vi "로봇대회1.vi"() -> ()   [LabVIEW 2010]
uses:
  <vilib>/NXT/Subs/MotorOutput.ctl
  <vilib>/NXT/Block Support/NXT_InputPort.ctl
  <vilib>/NXT/Dual Mode Library/Sensors/Sonar_cm.vi
  <vilib>/NXT/Dual Mode Library/Motors/MotorOn.vi
  <vilib>/NXT/Dual Mode Library/Sensors/Light_On.vi
  <vilib>/NXT/Dual Mode Library/Motors/MotorReverse.vi
  <vilib>/NXT/Dual Mode Library/Waits/Wait_Rotation.vi
  <vilib>/NXT/Dual Mode Library/Waits/Wait_Num.vi
panel:
  in  "정지":bool
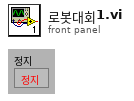
[diagram p1: front panel]
types:
  T1 = typedef "MotorOutput.ctl" = u8
  T2 = typedef "NXT_InputPort.ctl" = u8
  T3 = typedef "LVHSConnector.ctl" = cluster{"error":errorcluster, "address":string, "NXT #":i32, "Show Error":bool, "Connection":u16}
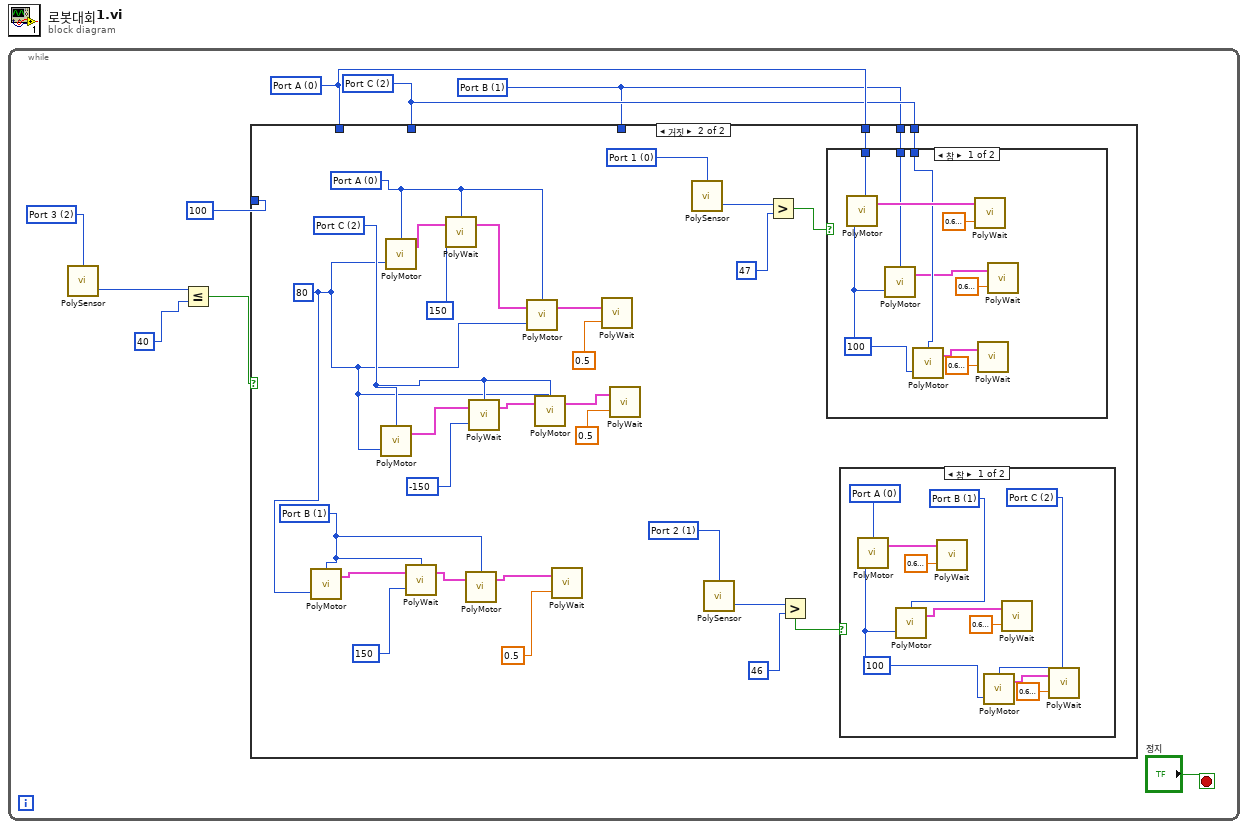
[diagram p0: block diagram]
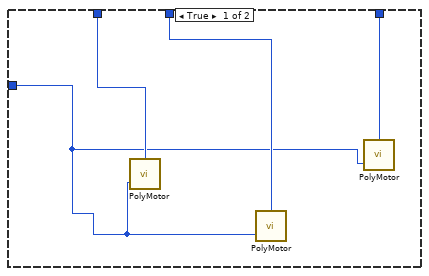
[diagram p2: hidden frame]
diagram:
  n1 = while {
    stop <- "정지" stop-if-true
    w1 = T1 1 items=["Port A", "Port B", "Port C", "All Ports"] ("Output Port (All Ports)")
    w2 = T1 2 items=["Port A", "Port B", "Port C", "All Ports"] ("Output Port (All Ports)")
    w3 = T1 0 items=["Port A", "Port B", "Port C", "All Ports"] ("Output Port (All Ports)")
    w6 = T2 2 items=["Port 1", "Port 2", "Port 3", "Port 4"] ("Input Port")
    n2 = call-poly <vilib>:"PolySensor.vi"("Port (Port 4)"=w6) -> ("Distance (cm)"=w4:i16)  [unwired: 2 in, 1 out]
    n3 = Less Or Equal?(x=w4, y=40) -> (x <= y?=w7:bool)
    n4 = case shown="거짓" w7 {
      tunnel: w3 -> [w13 _]
      tunnel: w2 -> [w12 _]
      tunnel: 100 ("Power (75)") -> [w10 _]
      tunnel: w1 -> [w11 _]
      tunnel: w3 -> [_ w23]
      tunnel: w2 -> [_ w22]
      tunnel: w1 -> [_ w21]
      frame True {
        n5 = call-poly <vilib>:"PolyMotor.vi"("Power (75)"=w10, "Output Port (All Ports)"=w13) -> ()  [unwired: 2 in, 1 out]
        n6 = call-poly <vilib>:"PolyMotor.vi"("Power (75)"=w10, "Output Port (All Ports)"=w12) -> ()  [unwired: 2 in, 1 out]
        n7 = call-poly <vilib>:"PolyMotor.vi"("Power (75)"=w10, "Output Port (All Ports)"=w11) -> ()  [unwired: 2 in, 1 out]
      }
      frame False {
        w14 = T1 1 items=["Port A", "Port B", "Port C", "All Ports"] ("Output Port (All Ports)")
        w25 = T2 1 items=["Port 1", "Port 2", "Port 3", "Port 4"] ("Input Port")
        w24 = T2 0 items=["Port 1", "Port 2", "Port 3", "Port 4"] ("Input Port")
        w17 = 80 ("Power (75)")
        w33 = T1 2 items=["Port A", "Port B", "Port C", "All Ports"] ("Output Port (All Ports)")
        w34 = T1 0 items=["Port A", "Port B", "Port C", "All Ports"] ("Output Port (All Ports)")
        n8 = call-poly <vilib>:"PolyMotor.vi"("Power (75)"=w17, "Output Port (All Ports)"=w14) -> ("NXT"=w18:T3)  [unwired: 2 in]
        n9 = call-poly <vilib>:"PolyMotor.vi"("Power (75)"=w17, "Output Port (All Ports)"=w33) -> ("NXT"=w42:T3)  [unwired: 2 in]
        n10 = call-poly <vilib>:"PolyMotor.vi"("Power (75)"=w17, "Output Port (All Ports)"=w34) -> ("NXT"=w43:T3)  [unwired: 2 in]
        n11 = call-poly <vilib>:"PolyWait.vi"("Position Change (180)"=150, "NXT"=w18, "Port (Port A)"=w14) -> ("NXT"=w19:T3)  [unwired: 1 in]
        n12 = call-poly <vilib>:"PolyWait.vi"("Position Change (180)"=150, "NXT"=w43, "Port (Port A)"=w34) -> ("NXT"=w39:T3)  [unwired: 1 in]
        n13 = call-poly <vilib>:"PolyMotor.vi"("NXT"=w19, "Output Port (All Ports)"=w14) -> ("NXT"=w20:T3)  [unwired: 2 in]
        n14 = call-poly <vilib>:"PolyWait.vi"("Position Change (180)"=-150, "NXT"=w42, "Port (Port A)"=w33) -> ("NXT"=w36:T3)  [unwired: 1 in]
        n15 = call-poly <vilib>:"PolyMotor.vi"("Power (75)"=w17, "NXT"=w39, "Output Port (All Ports)"=w34) -> ("NXT"=w38:T3)  [unwired: 1 in]
        n16 = call-poly <vilib>:"PolyMotor.vi"("Power (75)"=w17, "NXT"=w36, "Output Port (All Ports)"=w33) -> ("NXT"=w35:T3)  [unwired: 1 in]
        n17 = call-poly <vilib>:"PolyWait.vi"("Time (sec)"=sgl 0.5 ("Time (1 sec)"), "NXT"=w20) -> ()  [unwired: 2 in, 1 out]
        n18 = call-poly <vilib>:"PolyWait.vi"("Time (sec)"=sgl 0.5 ("Time (1 sec)"), "NXT"=w38) -> ()  [unwired: 2 in, 1 out]
        n19 = call-poly <vilib>:"PolyWait.vi"("Time (sec)"=sgl 0.5 ("Time (1 sec)"), "NXT"=w35) -> ()  [unwired: 2 in, 1 out]
        n20 = call-poly <vilib>:"PolySensor.vi"("Port (Port 3)"=w24) -> ("Scaled Value"=w28:i16)  [unwired: 2 in, 1 out]
        n21 = call-poly <vilib>:"PolySensor.vi"("Port (Port 3)"=w25) -> ("Scaled Value"=w31:i16)  [unwired: 2 in, 1 out]
        n22 = Greater?(x=w28, y=47) -> (0:w26:bool)
        n23 = Greater?(x=w31, y=46) -> (0:w29:bool)
        n24 = case shown="참" w26 {
          tunnel: w23 -> [w49 _]
          tunnel: w22 -> [w48 _]
          tunnel: w21 -> [w44 _]
          frame True {
            w45 = 100 ("Power (75)")
            n25 = call-poly <vilib>:"PolyMotor.vi"("Power (75)"=w45, "Output Port (All Ports)"=w49) -> ("NXT"=w53:T3)  [unwired: 2 in]
            n26 = call-poly <vilib>:"PolyMotor.vi"("Power (75)"=w45, "Output Port (All Ports)"=w44) -> ("NXT"=w46:T3)  [unwired: 2 in]
            n27 = call-poly <vilib>:"PolyMotor.vi"("Power (75)"=w45, "Output Port (All Ports)"=w48) -> ("NXT"=w52:T3)  [unwired: 2 in]
            n28 = call-poly <vilib>:"PolyWait.vi"("Time (sec)"=sgl 0.7, "NXT"=w53) -> ()  [unwired: 2 in, 1 out]
            n29 = call-poly <vilib>:"PolyWait.vi"("Time (sec)"=sgl 0.7, "NXT"=w52) -> ()  [unwired: 2 in, 1 out]
            n30 = call-poly <vilib>:"PolyWait.vi"("Time (sec)"=sgl 0.7, "NXT"=w46) -> ()  [unwired: 2 in, 1 out]
          }
          frame False {
          }
        }
        n31 = case shown="참" w29 {
          frame True {
            w55 = T1 1 items=["Port A", "Port B", "Port C", "All Ports"] ("Output Port (All Ports)")
            w58 = T1 2 items=["Port A", "Port B", "Port C", "All Ports"] ("Output Port (All Ports)")
            w59 = T1 0 items=["Port A", "Port B", "Port C", "All Ports"] ("Output Port (All Ports)")
            w54 = 100 ("Power (75)")
            n32 = call-poly <vilib>:"PolyMotor.vi"("Power (75)"=w54, "Output Port (All Ports)"=w59) -> ("NXT"=w63:T3)  [unwired: 2 in]
            n33 = call-poly <vilib>:"PolyMotor.vi"("Power (75)"=w54, "Output Port (All Ports)"=w55) -> ("NXT"=w56:T3)  [unwired: 2 in]
            n34 = call-poly <vilib>:"PolyWait.vi"("Time (sec)"=sgl 0.7, "NXT"=w63) -> ()  [unwired: 2 in, 1 out]
            n35 = call-poly <vilib>:"PolyMotor.vi"("Power (75)"=w54, "Output Port (All Ports)"=w58) -> ("NXT"=w62:T3)  [unwired: 2 in]
            n36 = call-poly <vilib>:"PolyWait.vi"("Time (sec)"=sgl 0.7, "NXT"=w56) -> ()  [unwired: 2 in, 1 out]
            n37 = call-poly <vilib>:"PolyWait.vi"("Time (sec)"=sgl 0.7, "NXT"=w62) -> ()  [unwired: 2 in, 1 out]
          }
          frame False {
          }
        }
      }
    }
  }
